vi "Write Data.vi"(10 "Data":i32, 11 "Feeder Task Msg in":refnum<class "Feeder Task Msg.lvclass">) -> (3 "Feeder Task Msg out":refnum<class "Feeder Task Msg.lvclass">)   [LabVIEW 2018, in "Feeder Task Msg.lvclass"]
uses:
  Feeder Task Msg.lvclass
  Feeder Task Msg.lvclass/Feeder Task Msg.ctl
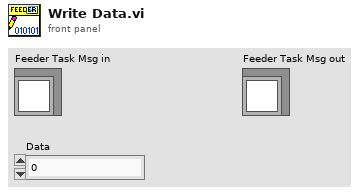
[diagram p1: front panel]
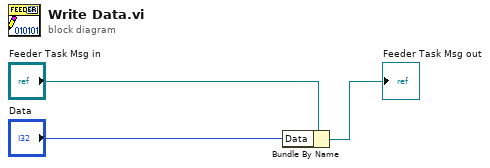
[diagram p0: block diagram]
diagram:
  n1 = Bundle By Name(cluster="Feeder Task Msg in", "Data"="Data") -> (→"Feeder Task Msg out":refnum<class "Feeder Task Msg.lvclass">)
